vi "cos_rise_tester.vi"() -> ()   [LabVIEW 2021]
uses:
  <instrlib>/_niInstr/Basic Elements/v1/FPGA/niInstr Basic Elements v1 FPGA.lvlib
panel:
  out "Waveform Chart 2":i16(graph)
  in  "stop":bool
  in  "t":fxp<+/-,16,1>=0.999969482421875
  out "x .or. y?":bool
  out "Waveform Chart":dbl(graph)
  out "data out":fxp<+/-,16,1>
  in  "change rate":u16
  in  "s":bool
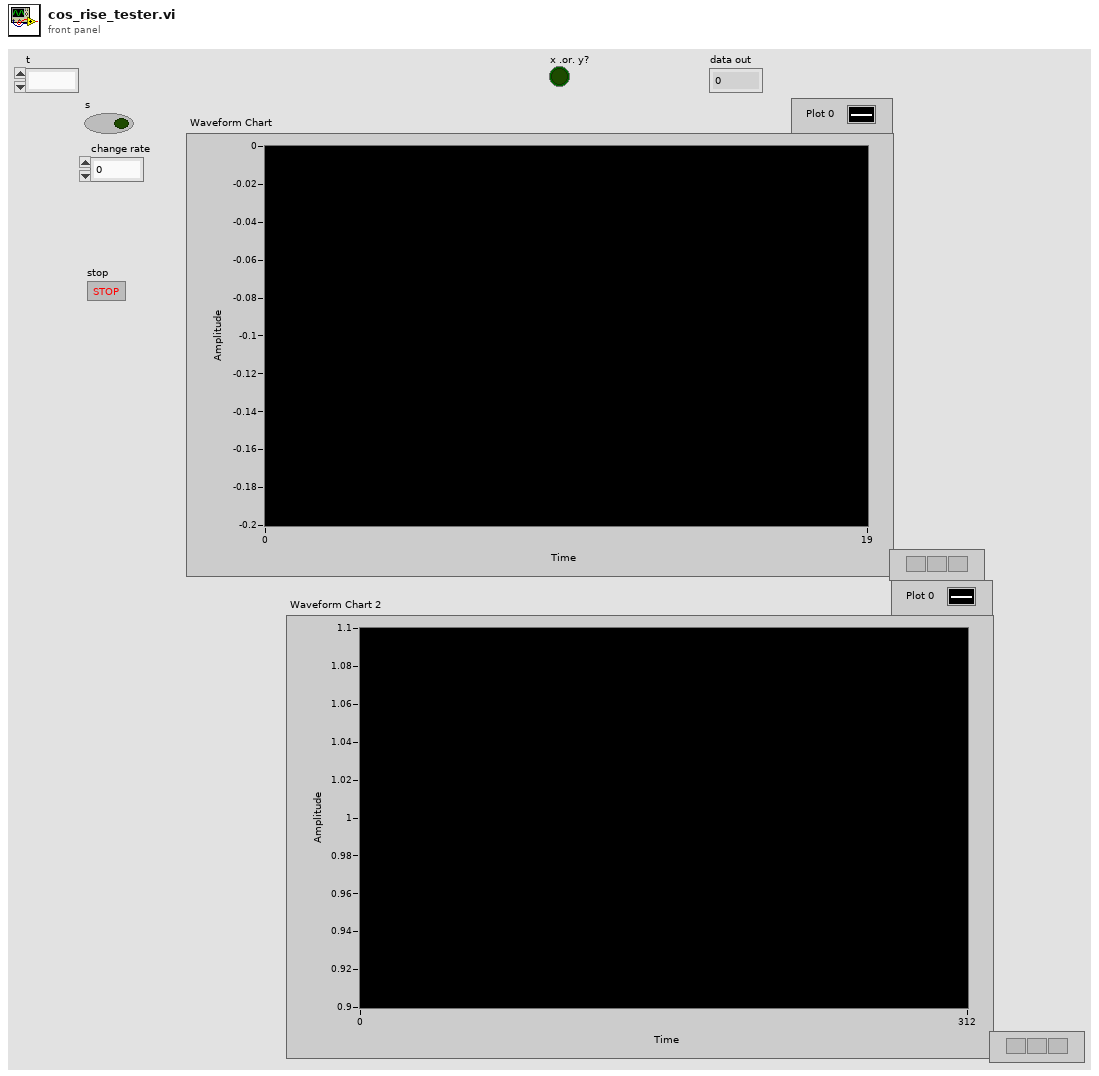
[diagram p1: front panel]
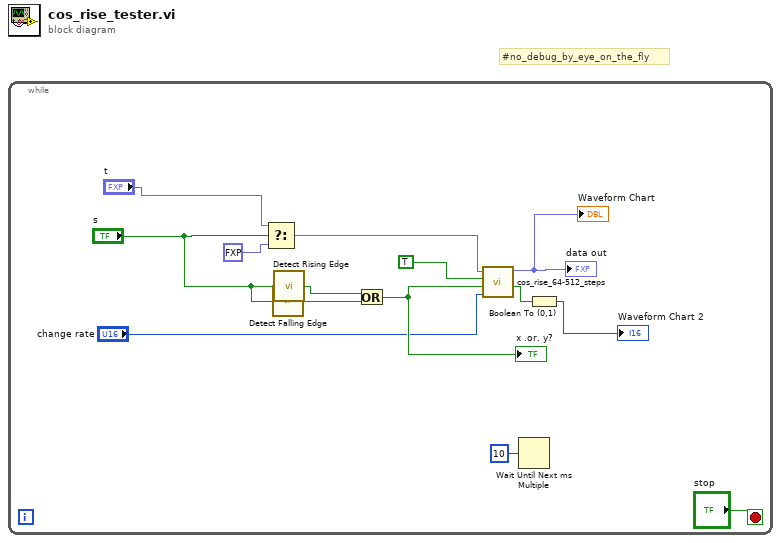
[diagram p0: block diagram]
diagram:
  # "#no_debug_by_eye_on_the_fly"
  n1 = while {
    stop <- "stop" stop-if-true
    n2 = Select(t="t", s="s", f=fxp<+/-,16,1> 0.0 ("data out")) -> (s? t:f=w14:fxp<+/-,16,1>)
    n3 = call <instrlib>:"Detect Falling Edge.vi"("signal"="s") -> ("edge detected"=w9:bool)  [unwired: 14 in]
    n4 = call <instrlib>:"Detect Rising Edge.vi"("signal"="s") -> ("edge detected"=w8:bool)  [unwired: 14 in]
    n5 = Or(x=w8, y=w9) -> (x .or. y?=w7:bool)
    "x .or. y?" <- w7
    n6 = call "cos_rise_64-512_steps.vi"("filter select"="change rate", "new step"=w7, "run"=TRUE, "data in"=w14) -> ("output valid"=w2:bool, "data out"=→"data out" →"Waveform Chart":fxp<+/-,16,1>)  [unwired: 5 in, 1 out]
    n7 = Wait Until Next ms Multiple(millisecond multiple=u32 10) -> ()  [unwired: 1 out]
    n8 = Boolean To (0,1)(Boolean=w2) -> (0, 1=→"Waveform Chart 2":i16)
  }
